vi "Configure IQ Adjustment External.vi"(0 "VISA resource name":refnum<visa-resource-name>, 1 "Differential Mode Q Offset (0 V)":dbl, 2 "Differential Mode I Offset (0 V)":dbl, 3 "Common Mode I/Q Offset (0 V)":dbl, 5 "External I Offset (0 V)":dbl, 7 "External Q Offset (0 V)":dbl, 9 "External Gain (0 dB)":dbl, 11 "error in (no error)":errorcluster, 12 "Attenuation Level (6 dB)":dbl=6.0, 13 "Quadrature Angle Adjustment (0 deg)":dbl) -> (4 "VISA resource name out":refnum<visa-resource-name>, 15 "error out":errorcluster)   [LabVIEW 2014, in "Agilent PSG MXG Series.lvlib"]
doc: "Configures external I/Q adjustments.\n\n<B>Notes:</B>\n(1) This VI is valid only in E8267C, E8267D, N5162A, N5182A, N5172B, N5182B.\n\n(2) For E8267C, this VI is valid only when the instrument installs <B>Option 002</B> (Internal baseband generator) or <B>Option 602</B> (Digital bus baseband generator)."
uses:
  Agilent PSG MXG Series.lvlib
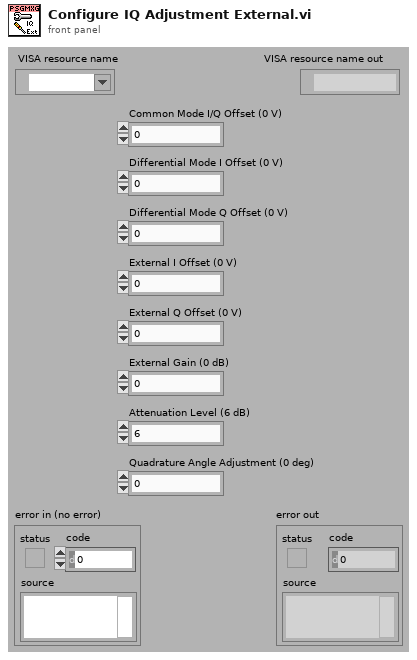
[diagram p1: front panel]
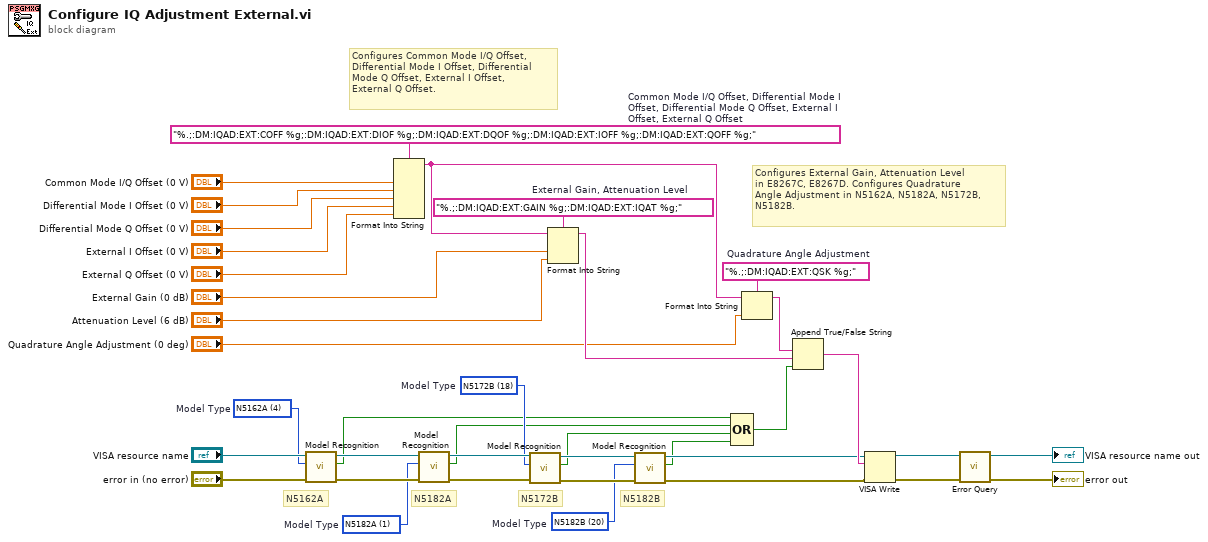
[diagram p0: block diagram]
diagram:
  w6 = u16 20 items=["N5181A"=0, "N5182A"=1, "N5183A"=2, "N5161A"=3, "N5162A"=4, "E8241A"=5, "E8244A"=6, "E8251A"=7, "E8254A"=8, "E8247C"=10, "E8257C"=11, "E8267C"=12, "E8257D"=15, "E8267D"=16, "N5171B"=17, "N5172B"=18, "N5181B"=19, "N5182B"=20]  # Model Type
  w7 = u16 18 items=["N5181A"=0, "N5182A"=1, "N5183A"=2, "N5161A"=3, "N5162A"=4, "E8241A"=5, "E8244A"=6, "E8251A"=7, "E8254A"=8, "E8247C"=10, "E8257C"=11, "E8267C"=12, "E8257D"=15, "E8267D"=16, "N5171B"=17, "N5172B"=18, "N5181B"=19, "N5182B"=20]  # Model Type
  w8 = u16 4 items=["N5181A"=0, "N5182A"=1, "N5183A"=2, "N5161A"=3, "N5162A"=4, "E8241A"=5, "E8244A"=6, "E8251A"=7, "E8254A"=8, "E8247C"=10, "E8257C"=11, "E8267C"=12, "E8257D"=15, "E8267D"=16, "N5171B"=17, "N5172B"=18, "N5181B"=19, "N5182B"=20]  # Model Type
  w9 = u16 1 items=["N5181A"=0, "N5182A"=1, "E8241A"=5, "E8244A"=6, "E8251A"=7, "E8254A"=8, "E8247C"=10, "E8257C"=11, "E8267C"=12, "E8257D"=15, "E8267D"=16]  # Model Type
  w27 = "%.;:DM:IQAD:EXT:QSK %g;"  # Quadrature Angle Adjustment
  w37 = "%.;:DM:IQAD:EXT:GAIN %g;:DM:IQAD:EXT:IQAT %g;"  # External Gain, Attenuation Level
  w38 = "%.;:DM:IQAD:EXT:COFF %g;:DM:IQAD:EXT:DIOF %g;:DM:IQAD:EXT:DQOF %g;:DM:IQAD:EXT:IOFF %g;:DM:IQAD:EXT:QOFF %g;"  # Common Mode I/Q Offset, Differential Mode I Offset, Differential Mode Q Offset, External I Offset, External Q Offset
  # "N5182B"
  # "N5172B"
  # "N5162A"
  # "Configures External Gain, Attenuation Level\nin E8267C, E8267D. Configures Quadrature\nAngle Adjustment in N5162A, N5182A, N5172B,\nN5182B."
  # "Configures Common Mode I/Q Offset,\nDifferential Mode I Offset, Differential\nMode Q Offset, External I Offset,\nExternal Q Offset."
  # "N5182A"
  n1 = call "Model Recognition.vi"("error in (no error)"="error in (no error)", "Model Type (0: N5181A)"=w8, "VISA resource name"="VISA resource name") -> ("error out"=w18:errorcluster, "Is Model Correct"=w2:bool, "VISA resource name out"=w14:refnum<visa-resource-name>)  [unwired: 6 out]
  n2 = Format Into String(format string=w38, "Common Mode I/Q Offset (0 V)", "Differential Mode I Offset (0 V)", "Differential Mode Q Offset (0 V)", "External I Offset (0 V)", "External Q Offset (0 V)") -> (resulting string=w28:string)  [unwired: 2 in, 1 out]
  n3 = call "Model Recognition.vi"("error in (no error)"=w18, "Model Type (0: N5181A)"=w9, "VISA resource name"=w14) -> ("error out"=w17:errorcluster, "Is Model Correct"=w3:bool, "VISA resource name out"=w13:refnum<visa-resource-name>)  [unwired: 6 out]
  n4 = call "Model Recognition.vi"("error in (no error)"=w17, "Model Type (0: N5181A)"=w7, "VISA resource name"=w13) -> ("error out"=w16:errorcluster, "Is Model Correct"=w4:bool, "VISA resource name out"=w12:refnum<visa-resource-name>)  [unwired: 6 out]
  n5 = Format Into String(format string=w37, initial string=w28, "External Gain (0 dB)", "Attenuation Level (6 dB)") -> (resulting string=w31:string)  [unwired: 1 in, 1 out]
  n6 = call "Model Recognition.vi"("error in (no error)"=w16, "Model Type (0: N5181A)"=w6, "VISA resource name"=w12) -> ("error out"=w10:errorcluster, "Is Model Correct"=w5:bool, "VISA resource name out"=w11:refnum<visa-resource-name>)  [unwired: 6 out]
  n7 = Compound Arithmetic op=OR(w2, w3, w4, w5) -> (w1:bool)
  n8 = Format Into String(format string=w27, initial string=w28, "Quadrature Angle Adjustment (0 deg)") -> (resulting string=w26:string)  [unwired: 1 in, 1 out]
  n9 = Append True/False String(1:w1, 2:w31, 3:w26) -> (0:w24:string)  [unwired: 1 out]
  n10 = VISA Write(VISA resource name=w11, write buffer=w24, error in (no error)=w10) -> (VISA resource name out=w23:refnum<visa-resource-name>, error out=w22:errorcluster)  [unwired: 1 out]
  n11 = call "Error Query.vi"("error in (no error)"=w22, "VISA resource name"=w23) -> ("error out"=→"error out":errorcluster, "VISA resource name out"=→"VISA resource name out":refnum<visa-resource-name>)  [unwired: 8 out]
